vi "AMWave.vi"() -> ()   [LabVIEW 2014]
uses:
  <vilib>/imath/engines/lvmath2/RunTimeEngine/Managers/WorkSpace/UID Generator.vi
  <vilib>/imath/engines/lvmath2/RunTimeEngine/RunTimeType/NIMS_RunTimeType_From StrictType (excl LVString).vi
  <instcachedir>/0/NIMS_RunTimeType_From StrictType (excl LVString)_15A5391EEA9C4AACB9955AC755B83D29.lvgen/NIMS_RunTimeType_From StrictType (excl LVString)_15A5391EEA9C4AACB9955AC755B83D29_000.vi
  <vilib>/imath/engines/lvmath2/RunTimeEngine/LocalVariableDefStatement/MC_LocalVariableDefStatement_Display.vi
  <vilib>/imath/engines/lvmath2/RunTimeEngine/RangeToken/NIMS_Range.vi
  <instcachedir>/0/NIMS_Range_9BCE657718DF4976A877346C61F22738.lvgen/NIMS_Range_9BCE657718DF4976A877346C61F22738_000.vi
  <vilib>/imathl/engines/lvmath/Functions/Error Handling/Create Error.vi
  <vilib>/imath/engines/lvmath2/RunTimeEngine/ArithmeticOperatorToken/NIMS_ArithmeticOperator_times.vi
  <instcachedir>/0/NIMS_ArithmeticOperator_times_2EFF5B13FCA4492A81D59089AD809F54.lvgen/NIMS_ArithmeticOperator_times_2EFF5B13FCA4492A81D59089AD809F54_000.vi
  <vilib>/imath/engines/lvmath2/RunTimeEngine/Managers/SymbolTable/Clear UID.vi
  <vilib>/imath/engines/lvmath2/RunTimeEngine/NodeEndStatement/NIMS_NodeEndStatement_Output.vi
  <instcachedir>/0/NIMS_NodeEndStatement_Output_53EC0D466D134D7ABD903AC30B43404B.lvgen/NIMS_NodeEndStatement_Output_53EC0D466D134D7ABD903AC30B43404B_005.vi
  <vilib>/imath/engines/lvmath2/RunTimeEngine/ErrorHandling/NIMS_Finalize Error.vi
  <vilib>/imath/engines/lvmath2/RunTimeEngine/Managers/SymbolTable/NIMS_WorkSpace.lvlib
panel:
  in  "AM Wave Parameters":T1 {"Amplitude" format="%#_13g"; "Modulation Frequency" format="%#_13g"; "Signal Frequency" format="%#_13g"}
  in  "Digitizing Parameters":T2 {"Sampling Frequency" format="%#_13g"; "Number of Samples" format="%#_13g"}
  out "AM Wave":cluster{"Time\n":dbl[], "Displacement":dbl[]}
  out "XY Graph":cluster{"t":dbl[], "d":dbl[]}(graph)
  # "Displays the AM Wave form with the given parameters."
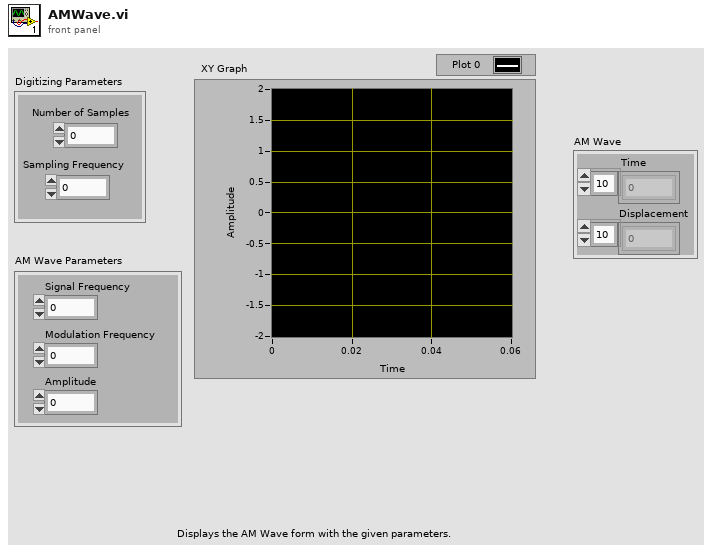
[diagram p1: front panel]
types:
  T1 = cluster{"Signal Frequency":dbl, "Modulation Frequency":dbl, "Amplitude":dbl}
  T2 = cluster{"Number of Samples":dbl, "Sampling Frequency":dbl}
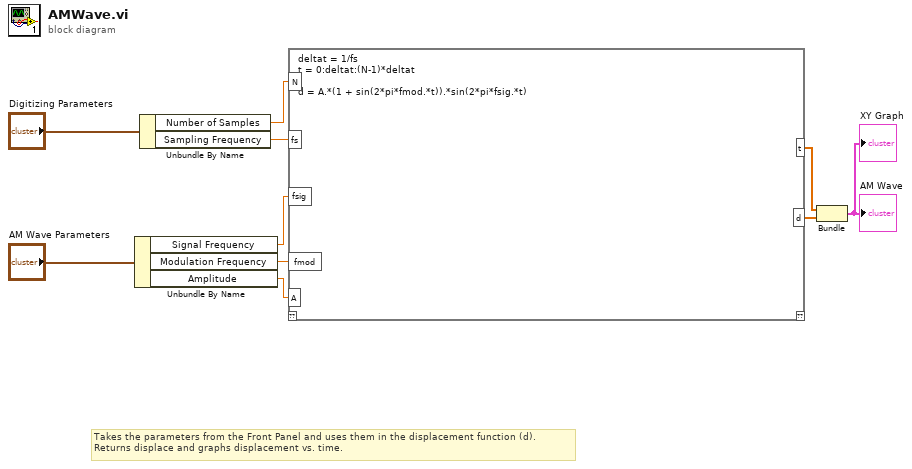
[diagram p0: block diagram]
diagram:
  # "Takes the parameters from the Front Panel and uses them in the displacement function (d).\nReturns displace and graphs displacement vs. time."
  n1 = Unbundle By Name("AM Wave Parameters") -> ("Signal Frequency"=w3:dbl, "Modulation Frequency"=w2:dbl, "Amplitude"=w1:dbl)
  n2 = Unbundle By Name("Digitizing Parameters") -> ("Number of Samples"=w5:dbl, "Sampling Frequency"=w4:dbl)
  n3 = mathscript code="deltat = 1/fs\nt = 0:deltat:(N-1)*deltat\n\nd = A.*(1 + sin(2*pi*fmod.*t)).*sin(2*pi*fsig.*t)"("N"=w5, "fs"=w4, "fsig"=w3, "fmod"=w2, "A"=w1) -> ("t"=w10:dbl[], "d"=w9:dbl[])  [unwired: 1 in, 1 out]
  n4 = Bundle("t"=w10, "d"=w9) -> (→"XY Graph" →"AM Wave":cluster{"t":dbl[], "d":dbl[]})  [unwired: 1 in]
